vi "Stream to Network.vi"() -> ()   [LabVIEW 2015]
uses:
  <vilib>/FPGAPlugInAG/cRIO-9063/niLvFpga_Open_cRIO-9063.vi
  <vilib>/rvi/interface/common/dynamic/niFpgaDynamicAddResources.vi
  <vilib>/Utility/error.llb/Error Cluster From Error Code.vi
  <vilib>/rvi/errors/niLvFpgaAdjustHostInterfaceError.vi
  <vilib>/FPGAPlugInAG/Dynamic/niLvFpga_Run_Dynamic.vi
  <vilib>/FPGAPlugInAG/Dynamic/niLvFpga_Close_Dynamic.vi
  <vilib>/rvi/interface/nirviOpenFPGA/nirviOpenFPGA.xnode
  FPGA Bitfiles/VCU-VEHICLEMODEL_FPGATarget_CANBasic(FPGA)_97RyJvtAznY.lvbitx
  Basic (FPGA) CAN Engine .vi
  <vilib>/rvi/interface/nirviMethod/nirviMethod.xnode
  <vilib>/rvi/interface/nirviReadWriteControl/nirviReadWriteControl.xnode
  <vilib>/rvi/interface/nirviCloseFPGA/nirviCloseFPGA.xnode
  <vilib>/rvi/errors/niLvFpgaMergeErrorWithErrorCode.vi
  <vilib>/rvi/interface/Simulation/niFpgaSimulationCallBeginRW.vi
  <vilib>/FPGAPlugInAG/Dynamic/niLvFpga_StartFifo_Dynamic.vi
  NiFpgaLv.dll
  <vilib>/FPGAPlugInAG/Dynamic/niLvFpga_ReadFifo_Dynamic.vi
panel:
  out "Overflow - Timed Out":bool
  in  "Stream":bool
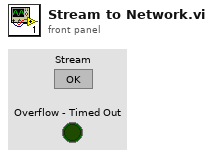
[diagram p1: front panel]
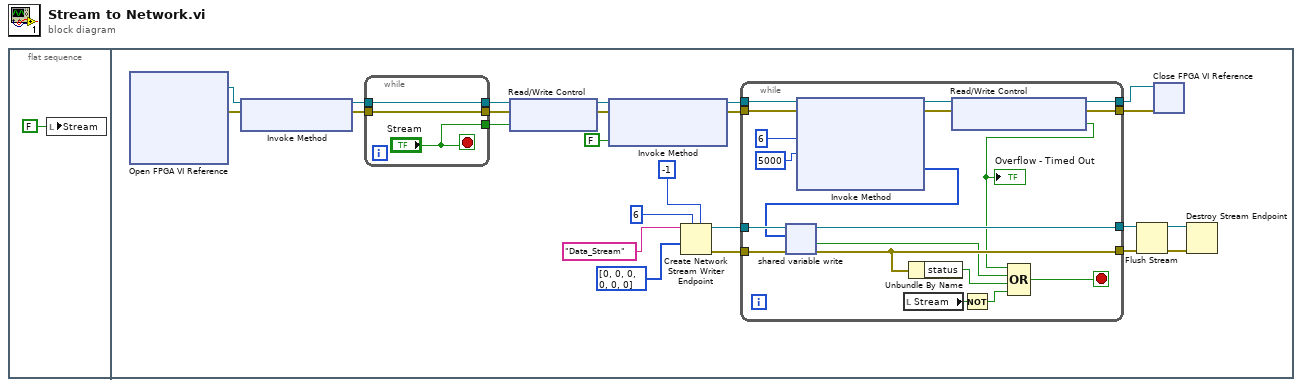
[diagram p0: block diagram]
diagram:
  n1 = flat-sequence {
    frame #0 {
      n2 = local write "Stream"(FALSE ("Stream")) -> ()
    }
    frame #1 {
      n3 = xnode "Open FPGA VI Reference"() -> ("FPGA VI Reference Out"=w11:refnum<k20>, "error out"=w12:errorcluster)  [unwired: 2 in]
      n4 = xnode "Invoke Method"("FPGA VI Reference In"=w11, "error in"=w12) -> ("FPGA VI Reference Out"=w10:refnum<k20>, "error out"=w9:errorcluster)
      n5 = while {
        tunnel: [w27] -> w25
        tunnel: [w28] -> w24
        tunnel: ["Stream"] -> w13
        tunnel: w10 -> [w28]
        tunnel: w9 -> [w27]
        stop <- "Stream" stop-if-true
      }
      n6 = xnode "Read/Write Control"("FPGA VI Reference In"=w24, "error in"=w25, "Log to buffer"=w13) -> ("FPGA VI Reference Out"=w8:refnum<k20>, "error out"=w6:errorcluster)
      n7 = xnode "Invoke Method"("FPGA VI Reference In"=w8, "error in"=w6, "Wait Until Done (F)"=FALSE) -> ("FPGA VI Reference Out"=w7:refnum<k20>, "error out"=w5:errorcluster)
      n8 = Create Network Stream Writer Endpoint(5:-1 ("timeout in ms (-1)"), 7:6 ("writer buffer size"), 9:u32[] [0, 0, 0, 0, 0, 0], 11:"Data_Stream" ("writer name")) -> (0:w20:errorcluster, 3:w21:refnum<k21>)  [unwired: 3 in]
      n9 = while {
        tunnel: w7 -> [w47]
        tunnel: w5 -> [w46]
        tunnel: [w42] -> w15
        tunnel: w21 -> [w43]
        tunnel: w20 -> [w40]
        tunnel: [w39] -> w17
        tunnel: [w37] -> w19
        tunnel: [w35] -> w18
        stop <- w33 stop-if-true
        n10 = xnode "Invoke Method"("FPGA VI Reference In"=w47, "error in"=w46, "Number of Elements"=u32 6, "Timeout (ms)"=5000) -> ("FPGA VI Reference Out"=w38:refnum<k20>, "error out"=w36:errorcluster, "Data"=w41:u32[])  [unwired: 1 out]
        n11 = shared-variable-write(w43, w40, w41) -> (w42:refnum<k21>, w39:errorcluster, w31:bool)  [unwired: 1 in]
        n12 = local read "Stream"() -> (w30:bool)
        n13 = Unbundle By Name(w39) -> ("status"=w34:bool)
        n14 = xnode "Read/Write Control"("FPGA VI Reference In"=w38, "error in"=w36) -> ("FPGA VI Reference Out"=w37:refnum<k20>, "error out"=w35:errorcluster, "Overflow - Timed Out"=w32:bool)
        "Overflow - Timed Out" <- w32
        n15 = Not(x=w30) -> (.not. x?=w29:bool)
        n16 = Compound Arithmetic op=OR(w32, w31, w34, w29) -> (w33:bool)
      }
      n17 = Flush Stream(8:w17, 11:w15) -> (0:w16:errorcluster, 3:w14:refnum<k21>)  [unwired: 2 in, 1 out]
      n18 = xnode "Close FPGA VI Reference"("FPGA VI Reference In"=w19, "error in"=w18) -> ()  [unwired: 1 out]
      n19 = Destroy Stream Endpoint(8:w16, 11:w14) -> ()  [unwired: 1 out]
    }
  }
